vi "Write All Variables.vi"(8 "error in (no error)":errorcluster, 10 "Config. vars.":T1, 11 "Config params in":refnum<class "CV-Configuration.lvclass">) -> (0 "error out":errorcluster, 3 "Config params out":refnum<class "CV-Configuration.lvclass">)   [LabVIEW 2013, in "CameraVision.lvlib" / "CV-Configuration.lvclass"]
uses:
  CV-Configuration.lvclass
  Configuration-variables.ctl
  Hardware/Camera/Camera.lvclass
  UI/Module-states.ctl
  CV-Configuration.lvclass/CV-Configuration.ctl
  UI/CV-UI.lvclass
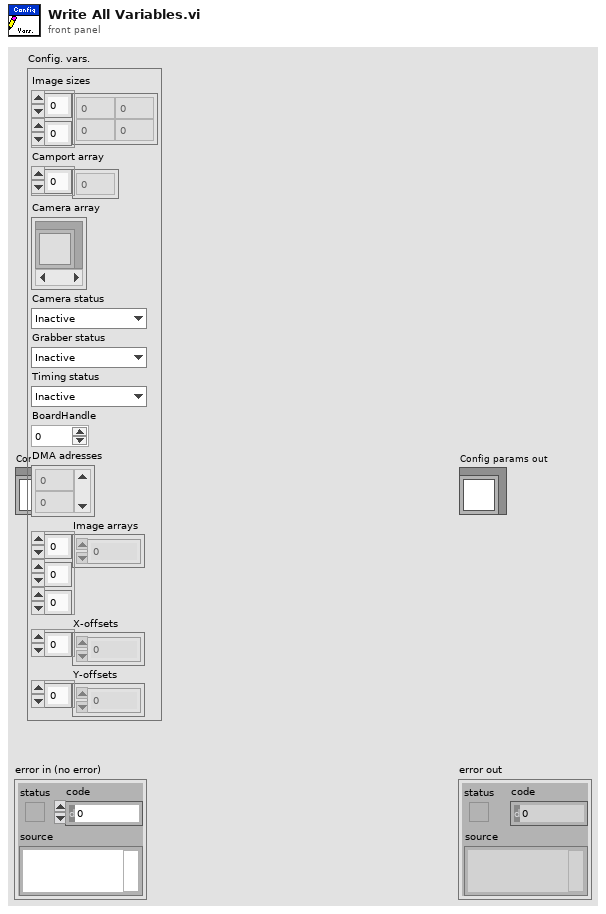
[diagram p1: front panel]
types:
  T1 = typedef "CameraVision.lvlib/CV-Configuration.lvclass/Configuration-variables.ctl" = cluster{"Image sizes":u32[][], "Camport array":u32[], "Camera array":refnum<class "Camera.lvclass">[], "Camera status":T2, "Grabber status":T2, "Timing status":T2, "BoardHandle":u64, "DMA adresses":i64[], "Image arrays":i8[][][], "X-offsets":i32[], "Y-offsets":i32[]}
  T2 = typedef "CameraVision.lvlib/CV-UI.lvclass/Module-states.ctl" = enum16{"Inactive", "Active", "Data-loss", "Error", "Simulation", "Synchronizing", "Initialized", "Released"}
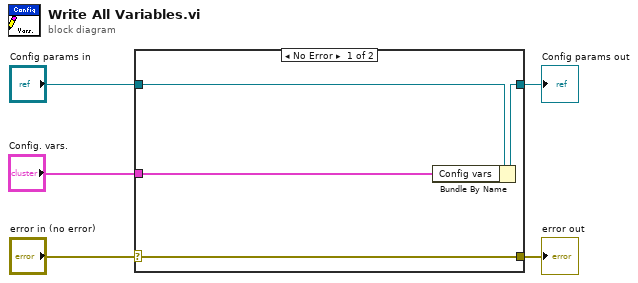
[diagram p0: block diagram]
diagram:
  n1 = case shown="No Error" "error in (no error)" {
    selector: "error in (no error)" -> [w9 w10]
    tunnel: [w9 w10] -> w4
    tunnel: [w7 w11] -> w2
    tunnel: "Config params in" -> [w8 w11]
    tunnel: "Config. vars." -> [w6 _]
    frame No Error {
      n2 = Bundle By Name(cluster=w8, "Config vars"=w6) -> (w7:refnum<class "CV-Configuration.lvclass">)
    }
    frame Error {
    }
  }
  "error out" <- w4
  "Config params out" <- w2
